vi "Main (10).vi"() -> ()   [LabVIEW 2018]
panel:
  in  "OK Button":bool
  in  "stop":bool
  out "LLenado":bool
  out "LLenado":bool
  out "Luz Baja 2":bool
  out "Luz Alta 2":bool
  in  "Dias Luz":string(combo)
  out "Unidades":string
  in  "Dias Temperatura":string(combo)
  in  "Centigrados":bool
  out "Intensidad  de Luz":u8(slide) scale=0.0..100.0
  out "Agua":dbl(slide) scale=0.0..200.0
  out "Comida":dbl(slide) scale=0.0..200.0
  out "Luz Baja":bool
  out "Luz Alta":bool
  out "Humedad":dbl(knob) scale=0.0..100.0
  out "H Baja":bool
  out "H Alta":bool
  out "T Baja":bool
  out "T Alta":bool
  out "Temperatura":dbl(slide) scale=0.0..100.0
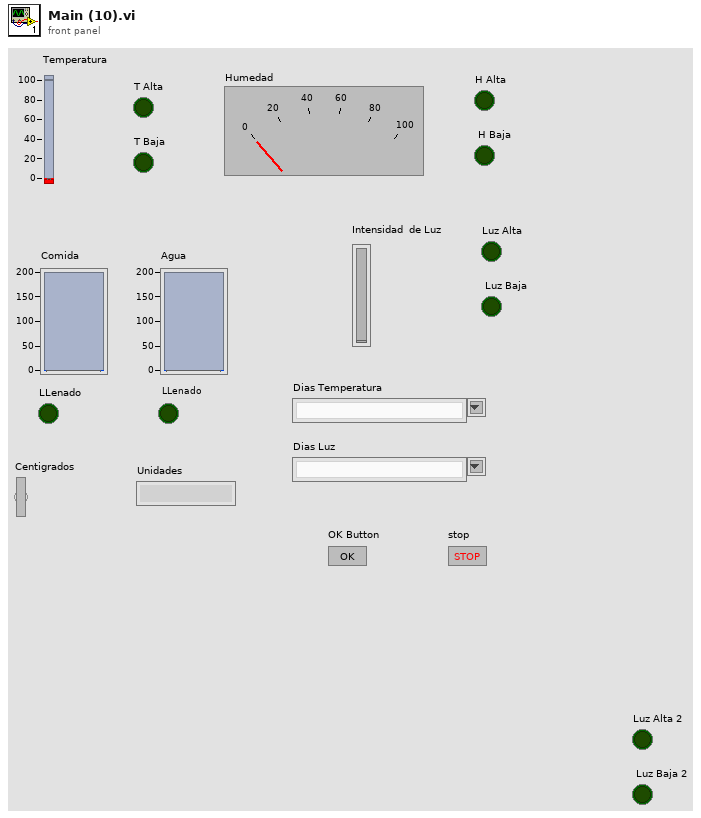
[diagram p1: front panel]
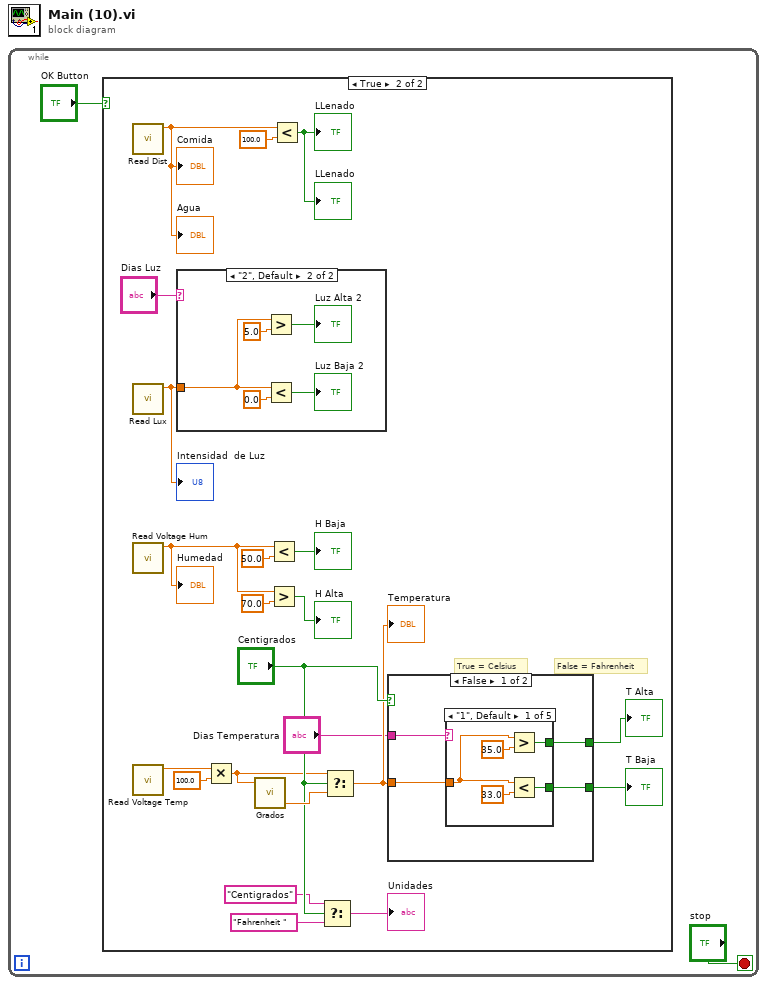
[diagram p0: block diagram]
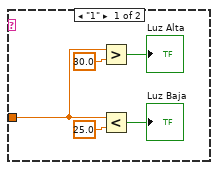
[diagram p3: hidden frame]
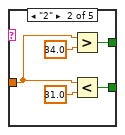
[diagram p4: hidden frame]
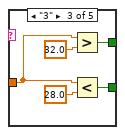
[diagram p5: hidden frame]
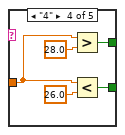
[diagram p6: hidden frame]
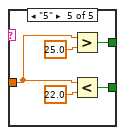
[diagram p7: hidden frame]
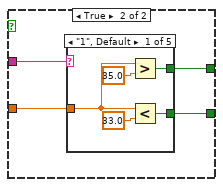
[diagram p8: hidden frame]
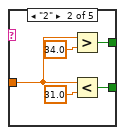
[diagram p9: hidden frame]
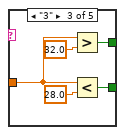
[diagram p10: hidden frame]
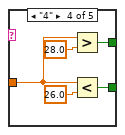
[diagram p11: hidden frame]
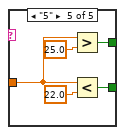
[diagram p12: hidden frame]
diagram:
  n1 = while {
    stop <- "stop" stop-if-true
    n2 = case shown="True" "OK Button" {
      frame False {
      }
      frame True {
        # "False = Fahrenheit"
        # "True = Celsius"
        n3 = call "Read Dist.vi"() -> ("distancia"=w14:dbl)  [unwired: 8 in, 1 out]
        "Comida" <- w14
        "Agua" <- w14
        n4 = call "Read Lux.vi"() -> ("lux"=w15:dbl)  [unwired: 8 in, 1 out]
        "Intensidad  de Luz" <- w15
        n5 = call "Read Voltage Hum.vi"() -> ("Porcentaje"=w17:dbl)  [unwired: 8 in, 1 out]
        "Humedad" <- w17
        n6 = call "Read Voltage Temp.vi"() -> ("Voltaje"=w21:dbl)  [unwired: 8 in, 1 out]
        n7 = case shown="\"2\", Default" "Dias Luz" {
          tunnel: w15 -> [w27 w30]
          frame "1" {
            n8 = Greater?(x=w27, y=30.0) -> (0:→"Luz Alta":bool)
            n9 = Less?(x=w27, y=25.0) -> (x < y?=→"Luz Baja":bool)
          }
          frame "2", Default {
            n10 = Greater?(x=w30, y=5.0) -> (0:→"Luz Alta 2":bool)
            n11 = Less?(x=w30, y=0.0) -> (x < y?=→"Luz Baja 2":bool)
          }
        }
        n12 = Multiply(x=w21, y=100.0) -> (x*y=w20:dbl)
        n13 = call "Grados.vi"("Grado"=w20) -> ("Conversion"=w23:dbl)  [unwired: 1 in]
        n14 = Less?(x=w17, y=50.0) -> (x < y?=→"H Baja":bool)
        n15 = Greater?(x=w17, y=70.0) -> (0:→"H Alta":bool)
        n16 = Less?(x=w14, y=100.0) -> (x < y?=→"LLenado" →"LLenado":bool)
        n17 = Select(t="Centigrados", s="Centigrados", f="Fahrenheit ") -> (s? t:f=→"Unidades":string)
        n18 = Select(t=w20, s="Centigrados", f=w23) -> (s? t:f=w12:dbl)
        "Temperatura" <- w12
        n19 = case shown="False" "Centigrados" {
          tunnel: w12 -> [w38 w67]
          tunnel: [w37 w66] -> w11
          tunnel: [w36 w65] -> w10
          tunnel: "Dias Temperatura" -> [w35 w64]
          frame False {
            n20 = case shown="\"1\", Default" w35 {
              tunnel: w38 -> [w41 w46 w51 w56 w61]
              tunnel: [w40 w45 w50 w55 w60] -> w37
              tunnel: [w39 w44 w49 w54 w59] -> w36
              frame "1", Default {
                n21 = Greater?(x=w41, y=35.0) -> (0:w40:bool)
                n22 = Less?(x=w41, y=33.0) -> (x < y?=w39:bool)
              }
              frame "2" {
                n23 = Greater?(x=w46, y=34.0) -> (0:w45:bool)
                n24 = Less?(x=w46, y=31.0) -> (x < y?=w44:bool)
              }
              frame "3" {
                n25 = Greater?(x=w51, y=32.0) -> (0:w50:bool)
                n26 = Less?(x=w51, y=28.0) -> (x < y?=w49:bool)
              }
              frame "4" {
                n27 = Greater?(x=w56, y=28.0) -> (0:w55:bool)
                n28 = Less?(x=w56, y=26.0) -> (x < y?=w54:bool)
              }
              frame "5" {
                n29 = Greater?(x=w61, y=25.0) -> (0:w60:bool)
                n30 = Less?(x=w61, y=22.0) -> (x < y?=w59:bool)
              }
            }
          }
          frame True {
            n31 = case shown="\"1\", Default" w64 {
              tunnel: w67 -> [w70 w75 w80 w85 w90]
              tunnel: [w69 w74 w79 w84 w89] -> w66
              tunnel: [w68 w73 w78 w83 w88] -> w65
              frame "1", Default {
                n32 = Greater?(x=w70, y=35.0) -> (0:w69:bool)
                n33 = Less?(x=w70, y=33.0) -> (x < y?=w68:bool)
              }
              frame "2" {
                n34 = Greater?(x=w75, y=34.0) -> (0:w74:bool)
                n35 = Less?(x=w75, y=31.0) -> (x < y?=w73:bool)
              }
              frame "3" {
                n36 = Greater?(x=w80, y=32.0) -> (0:w79:bool)
                n37 = Less?(x=w80, y=28.0) -> (x < y?=w78:bool)
              }
              frame "4" {
                n38 = Greater?(x=w85, y=28.0) -> (0:w84:bool)
                n39 = Less?(x=w85, y=26.0) -> (x < y?=w83:bool)
              }
              frame "5" {
                n40 = Greater?(x=w90, y=25.0) -> (0:w89:bool)
                n41 = Less?(x=w90, y=22.0) -> (x < y?=w88:bool)
              }
            }
          }
        }
        "T Baja" <- w10
        "T Alta" <- w11
      }
    }
  }
